vi "LinDaten Index.vi"(9 "Messbereich":u16, 11 "Komponente":u16) -> (0 "Index Analysator":u16, 1 "Index Komponente":u16, 3 "Index Lin":u16)   [LabVIEW 2015, in "Linearisierung v2.lvlib" / "Gasteiler.lvlib"]
uses:
  Gasteiler.lvlib
  Seiten/FT-IR/FT-IR.lvlib
  Seiten/FT-IR/FGV FT-IR Gasliste Aktionen.ctl
  Seiten/FT-IR/Algebraic Modul/Algebraic Modul.lvlib
  Seiten/FT-IR/Algebraic Modul/FGV Algebraic Aktionen.ctl
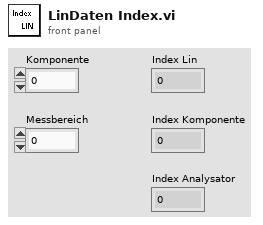
[diagram p1: front panel]
types:
  T1 = typedef "FT-IR.lvlib/Algebraic Modul.lvlib/FGV Algebraic Aktionen.ctl" = enum16{"lesen", "laden", "speichern", "berechnen", "schreiben"}
  T2 = typedef "FT-IR.lvlib/FGV FT-IR Gasliste Aktionen.ctl" = enum16{"lesen", "Gasliste FT-IR", "Gasliste ausgelesen", "laden", "speichern", "löschen"}
  T3 = typedef "String - Ausgabefeld.ctl" = string
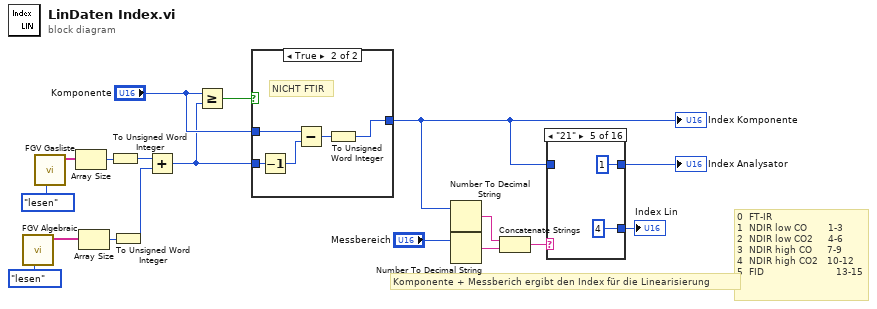
[diagram p0: block diagram]
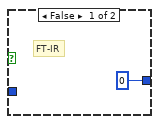
[diagram p2: hidden frame]
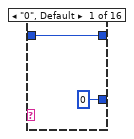
[diagram p3: hidden frame]
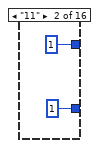
[diagram p4: hidden frame]
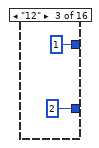
[diagram p5: hidden frame]
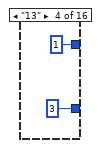
[diagram p6: hidden frame]
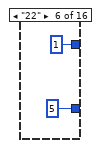
[diagram p7: hidden frame]
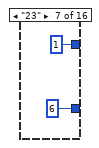
[diagram p8: hidden frame]
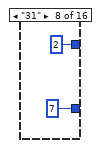
[diagram p9: hidden frame]
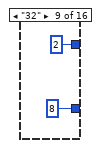
[diagram p10: hidden frame]
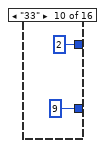
[diagram p11: hidden frame]
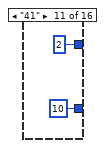
[diagram p12: hidden frame]
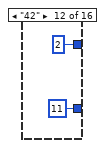
[diagram p13: hidden frame]
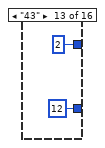
[diagram p14: hidden frame]
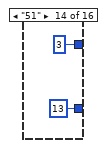
[diagram p15: hidden frame]
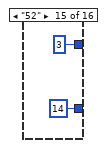
[diagram p16: hidden frame]
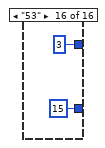
[diagram p17: hidden frame]
diagram:
  # "0  FT-IR\n1  NDIR low CO       1-3\n2  NDIR low CO2     4-6\n3  NDIR high CO     7-9\n4  NDIR high CO2   10-12\n5  FID                        13-15"
  # "Komponente + Messberich ergibt den Index für die Linearisierung"
  n1 = call "FGV Algebraic.vi"("Aktionen Algebraic"=FGV_Algebraic_Aktionen."lesen") -> ("Namen"=w4:string[])  [unwired: 6 in, 4 out]
  n2 = call "FGV Gasliste.vi"("Aktionen"=FGV_FT-IR_Gasliste_Aktionen."lesen") -> ("Aktuelle Gasliste FT-IR"=w13:T3[])  [unwired: 8 in, 2 out]
  n3 = Array Size(array=w13) -> (size(s)=w11:i32)
  n4 = Array Size(array=w4) -> (size(s)=w5:i32)
  n5 = To Unsigned Word Integer(number=w11) -> (unsigned 16bit integer=w3:u16)
  n6 = To Unsigned Word Integer(number=w5) -> (unsigned 16bit integer=w2:u16)
  n7 = Add(x=w3, y=w2) -> (x+y=w1:u16)
  n8 = Greater Or Equal?(x="Komponente", y=w1) -> (x >= y?=w12:bool)
  n9 = case shown="True" w12 {
    tunnel: "Komponente" -> [_ w24]
    tunnel: w1 -> [_ w23]
    tunnel: [u16 0 w20] -> w6
    frame False {
      # "FT-IR"
    }
    frame True {
      # "NICHT FTIR"
      n10 = Decrement(x=w23) -> (x-1=w22:u16)
      n11 = Subtract(x=w24, y=w22) -> (x-y=w21:u16)
      n12 = To Unsigned Word Integer(number=w21) -> (unsigned 16bit integer=w20:u16)
    }
  }
  "Index Komponente" <- w6
  n13 = Number To Decimal String(number=w6) -> (decimal integer string=w18:string)  [unwired: 1 in]
  n14 = Number To Decimal String(number="Messbereich") -> (decimal integer string=w17:string)  [unwired: 1 in]
  n15 = Concatenate Strings(w18, w17) -> (w16:string)
  n16 = case shown="\"21\"" w16 {
    tunnel: [u16 0 u16 1 u16 2 u16 3 u16 4 u16 5 u16 6 u16 7 u16 8 u16 9 u16 10 u16 11 u16 12 u16 13 u16 14 u16 15] -> w14
    tunnel: w6 -> [w25 _ _ _ _ _ _ _ _ _ _ _ _ _ _ _]
    tunnel: [w25 u16 1 u16 1 u16 1 u16 1 u16 1 u16 1 u16 2 u16 2 u16 2 u16 2 u16 2 u16 2 u16 3 u16 3 u16 3] -> w8
    frame "0", Default {
    }
    frame "11" {
    }
    frame "12" {
    }
    frame "13" {
    }
    frame "21" {
    }
    frame "22" {
    }
    frame "23" {
    }
    frame "31" {
    }
    frame "32" {
    }
    frame "33" {
    }
    frame "41" {
    }
    frame "42" {
    }
    frame "43" {
    }
    frame "51" {
    }
    frame "52" {
    }
    frame "53" {
    }
  }
  "Index Lin" <- w14
  "Index Analysator" <- w8
